vi "parse_string.vi"(11 "Input":string) -> (2 "Argument":string, 3 "Stanje":string)   [LabVIEW 2023]
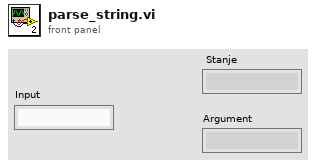
[diagram p1: front panel]
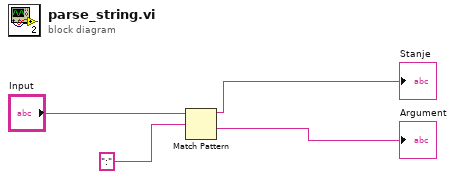
[diagram p0: block diagram]
diagram:
  n1 = Match Pattern(string="Input", regular expression=":") -> (before substring=→"Stanje":string, after substring=→"Argument":string)  [unwired: 1 in, 2 out]
